vi "Get CSV Header.vi"(8 "error in (no error)":errorcluster, 11 "Trace in":refnum<class "Trace.lvclass">) -> (0 "error out":errorcluster, 2 "CSV Header":string, 3 "Trace out":refnum<class "Trace.lvclass">)   [LabVIEW 2014, in "Robot Actor Framework.lvlib" / "Trace.lvlib" / "Trace.lvclass"]
uses:
  Trace.lvclass
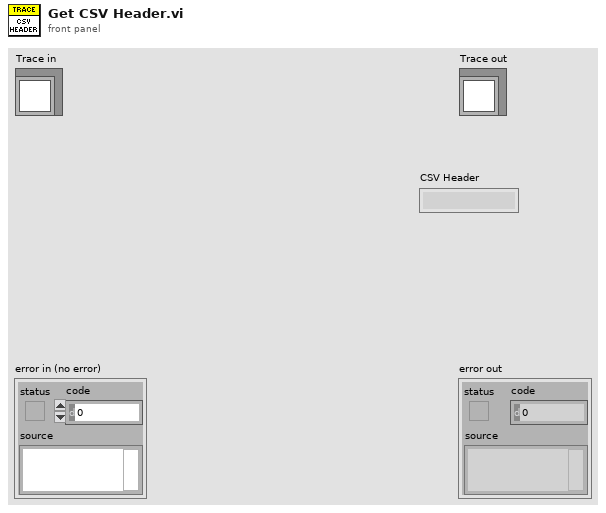
[diagram p1: front panel]
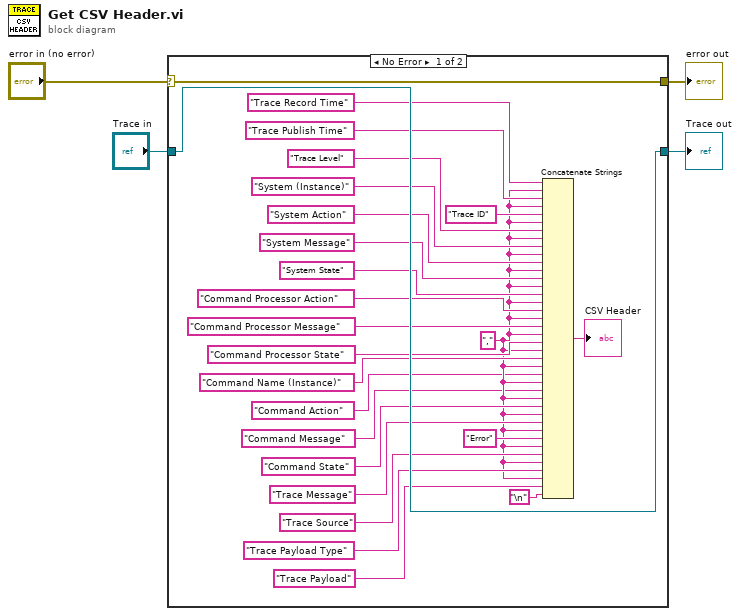
[diagram p0: block diagram]
diagram:
  n1 = case shown="No Error" "error in (no error)" {
    selector: "error in (no error)" -> [w28 w31]
    tunnel: [w28 w31] -> w3
    tunnel: [w29 w30] -> w1
    tunnel: "Trace in" -> [w29 w30]
    frame No Error {
      w7 = "," ("string")
      n2 = Concatenate Strings("Trace Record Time" ("string"), w7, "Trace Publish Time" ("string"), w7, "Trace ID" ("string"), w7, "Trace Level" ("string"), w7, "System (Instance)" ("string"), w7, "System Action" ("string"), w7, "System Message" ("string"), w7, "System State" ("string"), w7, "Command Processor Action" ("string"), w7, "Command Processor Message" ("string"), w7, "Command Processor State" ("string"), w7, "Command Name (Instance)" ("string"), w7, "Command Action" ("string"), w7, "Command Message" ("string"), w7, "Command State" ("string"), w7, "Trace Message" ("string"), w7, "Error" ("string"), w7, "Trace Source" ("string"), w7, "Trace Payload Type" ("string"), w7, "Trace Payload" ("string"), "\n") -> (→"CSV Header":string)
    }
    frame Error {
    }
  }
  "error out" <- w3
  "Trace out" <- w1
